vi "jsonParseBool.vi"(8 "error in (no error)":errorcluster, 9 "default":bool, 10 "path":string, 11 "d in":i64) -> (0 "error out":errorcluster, 1 "found?":bool, 2 "value":bool, 3 "d out":i64)   [LabVIEW 2015, in "rapidjson wrapper.lvlib"]
uses:
  rapidjson wrapper.lvlib
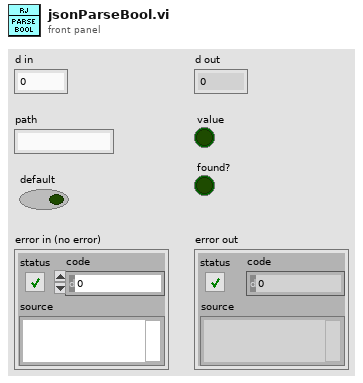
[diagram p1: front panel]
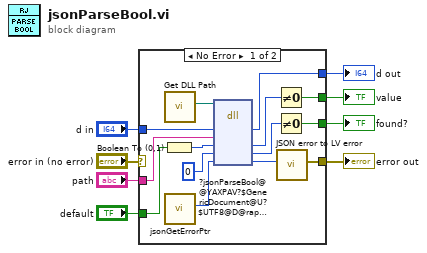
[diagram p0: block diagram]
diagram:
  n1 = case shown="No Error" "error in (no error)" {
    selector: "error in (no error)" -> [_ w25]
    tunnel: [w20 w25] -> w8
    tunnel: [w17 w24] -> w6
    tunnel: "default" -> [w16 w24]
    tunnel: "d in" -> [w15 w23]
    tunnel: "path" -> [w14 _]
    tunnel: [w13 w23] -> w2
    tunnel: [w9 _] -> w1
    frame No Error {
      n2 = Boolean To (0,1)(Boolean=w16) -> (0, 1=w18:i16)
      n3 = call "Get DLL Path.vi"() -> ("Path"=w22:path)  [unwired: 11 in]
      n4 = call "jsonGetErrorPtr.vi"() -> ("return type"=w19:i64)  [unwired: 10 in, 1 out]
      n5 = dll-call lib="C:/Users/tblair/Documents/Git Projects/rapidjson-for-LabVIEW/lvrjs/Debug/lvrjs.dll" fn="?jsonParseBool@@YAXPAV?$GenericDocument@U?$UTF8@D@rapidjson@@V?$MemoryPoolAllocator@VCrtAllocator@rapidjson@@@2@VCrtAllocator@2@@rapidjson@@PADAA_N20@Z"(path in=w22, "d"=w15, "path"=w14, "value"=w18, "replaced"=0, "jsonError"=w19) -> ("d"=w13:i64, "value"=w10:i32, "replaced"=w11:i32, "jsonError"=w21:i64)  [unwired: 4 in, 2 out]
      n6 = Not Equal To 0?(x=w10) -> (x != 0?=w17:bool)
      n7 = Not Equal To 0?(x=w11) -> (x != 0?=w9:bool)
      n8 = call "JSON error to LV error.vi"("jsonError"=w21) -> ("error out"=w20:errorcluster)  [unwired: 10 in]
    }
    frame Error {
    }
  }
  "error out" <- w8
  "value" <- w6
  "d out" <- w2
  "found?" <- w1
